vi "LVClass_SlopesPostProcessList AddProcessor_Modulator.vi"(0 "SlopesPostProcessorList in":refnum<class "SlopesPostProcessorList.lvclass">, 5 "Position":i32, 7 "Modulator":T1, 11 "error in (no error)":errorcluster) -> (4 "SlopesPostProcessorList out":refnum<class "SlopesPostProcessorList.lvclass">, 15 "error out":errorcluster)   [LabVIEW 2020, in "SlopesPostProcessorList.lvclass"]
doc: "Insert a Filter processor.\n\n--------------------------------------------------------------------------------\n\n<B>SlopesPostProcessorListIn </B> : SlopesPostProcessorList object.\n<B>SlopesPostProcessorListOut </B> : SlopesPostProcessorList object.\n<B>position </B> : Position of the processor in the SlopesPostProcessorList.\n<B>apply_tiltx_filter </B> : Activate x tilt filter.\n<B>apply_tilty_filter </B> : Activate y tilt filter.\n<B>apply_curv_filter </B> : Activate curvature filter.\n<B>apply_astig0_filter </B> : Activate 0 degree astigmatism filter.\n<B>apply_astig45_filter </B> : Activate 45 degree astigmatism filter.\n<B>apply_others_filter </B> : Activate all other aberrations filter.\n<B>ErrorIn </B> : Error\n<B>ErrorOut </B> : Error\n\n--------------------------------------------------------------------------------"
uses:
  SlopesPostProcessorList.lvclass
  SlopesPostProcessorList - Modulator.ctl
  SlopesPostProcessorList.lvclass/SlopesPostProcessorList.ctl
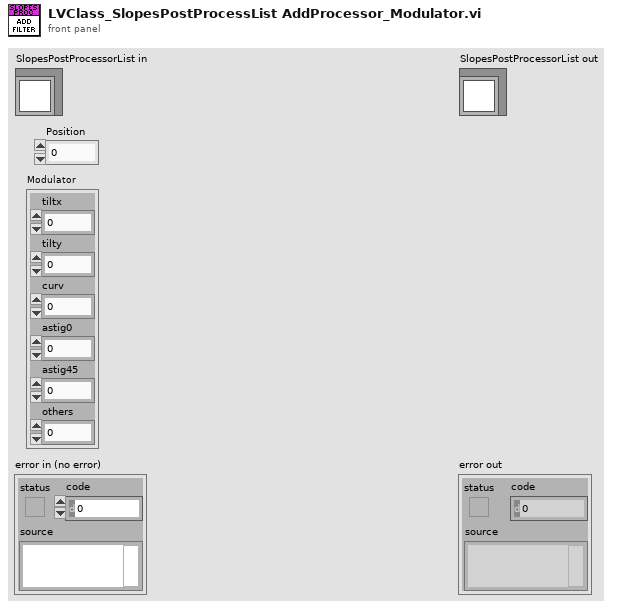
[diagram p1: front panel]
types:
  T1 = typedef "SlopesPostProcessorList - Modulator.ctl" = cluster{"tiltx":sgl, "tilty":sgl, "curv":sgl, "astig0":sgl, "astig45":sgl, "others":sgl}
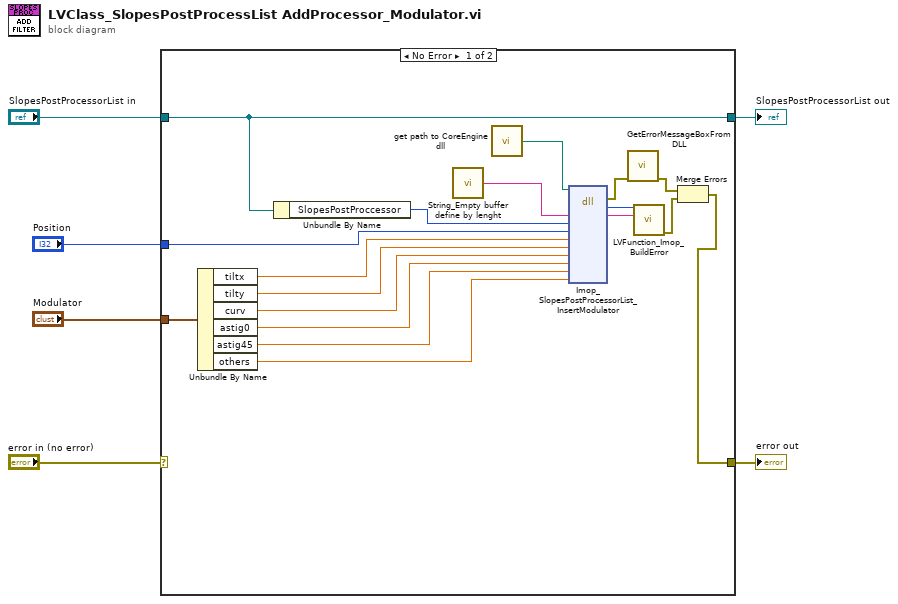
[diagram p0: block diagram]
diagram:
  n1 = case shown="No Error" "error in (no error)" {
    selector: "error in (no error)" -> [_ w26]
    tunnel: [w14 w26] -> w5
    tunnel: [w19 w25] -> w3
    tunnel: "SlopesPostProcessorList in" -> [w19 w25]
    tunnel: "Modulator" -> [w17 _]
    tunnel: "Position" -> [w13 _]
    frame No Error {
      n2 = Unbundle By Name(w17) -> ("tiltx"=w12:sgl, "tilty"=w11:sgl, "curv"=w10:sgl, "astig0"=w9:sgl, "astig45"=w8:sgl, "others"=w7:sgl)
      n3 = Unbundle By Name(w19) -> ("SlopesPostProccessor"=w18:i32)
      n4 = call "String_Empty buffer define by lenght.vi"() -> ("Empty buffer"=w24:string)  [unwired: 1 in]
      n5 = call "get path to CoreEngine dll.vi"() -> ("path to c_interface_vc100.dll"=w21:path)  [unwired: 12 in, 3 out]
      n6 = dll-call lib="D:/soft/HASO_v3/SVN_trunk/ImOpCoreEngine4_LV2011/DLLs/c_interface_vc100.dll" fn="Imop_SlopesPostProcessorList_InsertModulator"(path in=w21, "message"=w24, "objet"=w18, "Position"=w13, "tiltX"=w12, "tiltY"=w11, "Curv"=w10, "Astig0"=w9, "Astig45"=w8, "others"=w7) -> (error out=w20:errorcluster, "return type"=w22:i32, "message"=w23:string)  [unwired: 10 in, 1 out]
      n7 = call "GetErrorMessageBoxFromDLL.vi"("error IN"=w20) -> ("error OUT"=w16:errorcluster)  [unwired: 10 in]
      n8 = call "LVFunction_Imop_BuildError.vi"("code"=w22, "String to Prepend to source (\"\")"=w23) -> ("error out"=w15:errorcluster)  [unwired: 13 in]
      n9 = Merge Errors(w16, w15) -> (w14:errorcluster)
    }
    frame Error {
    }
  }
  "error out" <- w5
  "SlopesPostProcessorList out" <- w3
